vi "TestExec.Script Split Address and Function.vi"(8 "error in":errorcluster, 11 "string":string) -> (0 "error out":errorcluster, 2 "Funct":string, 3 "Addr":string)   [LabVIEW 2017]
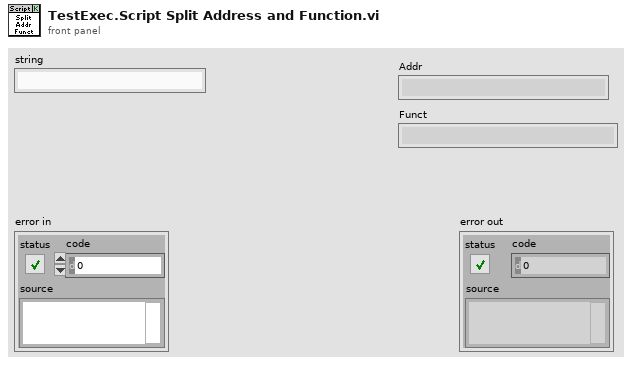
[diagram p1: front panel]
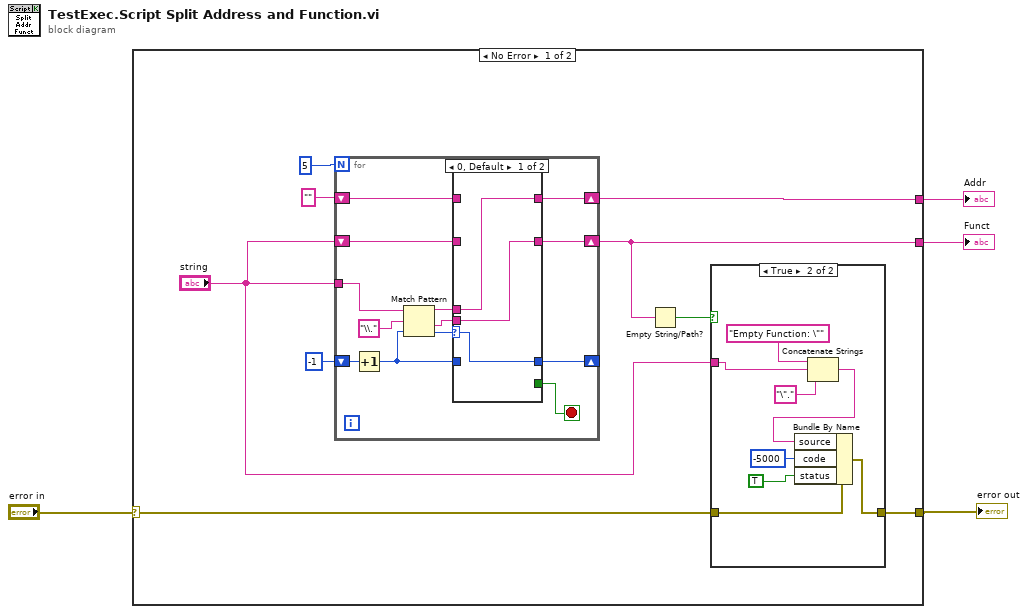
[diagram p0: block diagram]
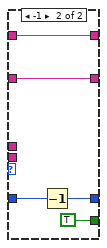
[diagram p3: hidden frame]
diagram:
  n1 = case shown="No Error" "error in" {
    selector: "error in" -> [w6 w43]
    tunnel: [w11 _] -> w4
    tunnel: [w9 _] -> w3
    tunnel: [w5 w43] -> w1
    frame No Error {
      n2 = for {
        N: 5 -> [_]
        tunnel: "string" -> [w33]
        shift-right: [w31] -> _
        shift-left: -1 -> [w30]
        shift-right: [w23] -> w11
        shift-left: "" -> [w25]
        shift-right: [w22] -> w9
        shift-left: "string" -> [w24]
        stop <- w26 stop-if-true
        n3 = Increment(x=w30) -> (x+1=w29:i32)
        n4 = Match Pattern(string=w33, regular expression="\\.", offset (0)=w29) -> (before substring=w28:string, after substring=w27:string, offset past match=w32:i32)  [unwired: 1 out]
        n5 = case shown="0, Default" w32 {
          selector: w32 -> [w37 _]
          tunnel: w29 -> [_ w41]
          tunnel: [w37 w42] -> w31
          tunnel: w28 -> [w36 _]
          tunnel: w27 -> [w35 _]
          tunnel: [_ TRUE] -> w26
          tunnel: w25 -> [_ w39]
          tunnel: w24 -> [_ w38]
          tunnel: [w36 w39] -> w23
          tunnel: [w35 w38] -> w22
          frame 0, Default {
          }
          frame -1 {
            n6 = Decrement(x=w41) -> (x-1=w42:i32)
          }
        }
      }
      n7 = Empty String/Path?(string/path=w9) -> (empty?=w8:bool)
      n8 = case shown="True" w8 {
        tunnel: "string" -> [_ w15]
        tunnel: w6 -> [_ w21]
        tunnel: [_ w20] -> w5
        frame False {
        }
        frame True {
          n9 = Concatenate Strings("Empty Function: \"", w15, "\".") -> (w14:string)
          n10 = Bundle By Name(cluster=w21, "source"=w14, "code"=-5000, "status"=TRUE) -> (w20:errorcluster)
        }
      }
    }
    frame Error {
    }
  }
  "Addr" <- w4
  "Funct" <- w3
  "error out" <- w1
